vi "Update_Attribute_Tree_POLARIS.vi"(4 "Flush Tree?":bool, 5 "error in":errorcluster, 6 "Filter":string, 7 "Tree Control In":refnum<vi>, 8 "Attribute Information Array":T1[](array[typedef])) -> (0 "error out":errorcluster)   [LabVIEW 2020, in "Camera Settings Dialog UI.lvlib" / "Camera Settings Dialog.lvclass"]
doc: "The Update Attribute Tree subVI, enumerates the attributes available for the camera and populates the Attribute Tree control with the attribute list."
uses:
  Camera Settings Dialog.lvclass
  Camera Attribute Info.ctl
  Camera Settings Dialog.lvclass/Camera Settings Dialog.ctl
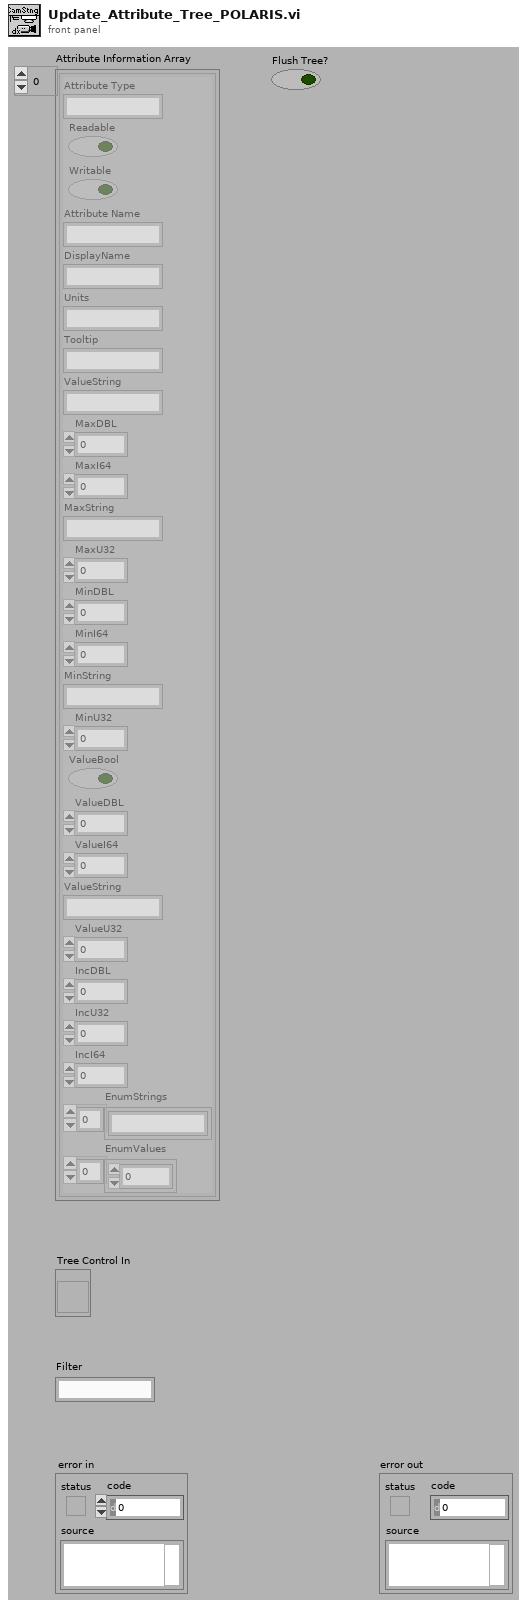
[diagram p1: front panel]
types:
  T1 = typedef "Camera Attribute Info.ctl" = cluster{"Attribute Type":string, "Readable":bool, "Writable":bool, "Attribute Name":string, "DisplayName":string, "Units":string, "Tooltip":string, "ValueString":string, "MaxDBL":dbl, "MaxI64":i64, "MaxString":string, "MaxU32":u32, "MinDBL":dbl, "MinI64":i64, "MinString":string, "MinU32":u32, "ValueBool":bool, "ValueDBL":dbl, "ValueI64 ":i64, "ValueString":string, "ValueU32":u32, "IncDBL":dbl, "IncU32":u32, "IncI64":i64, "EnumStrings":string[], "EnumValues":u32[]}
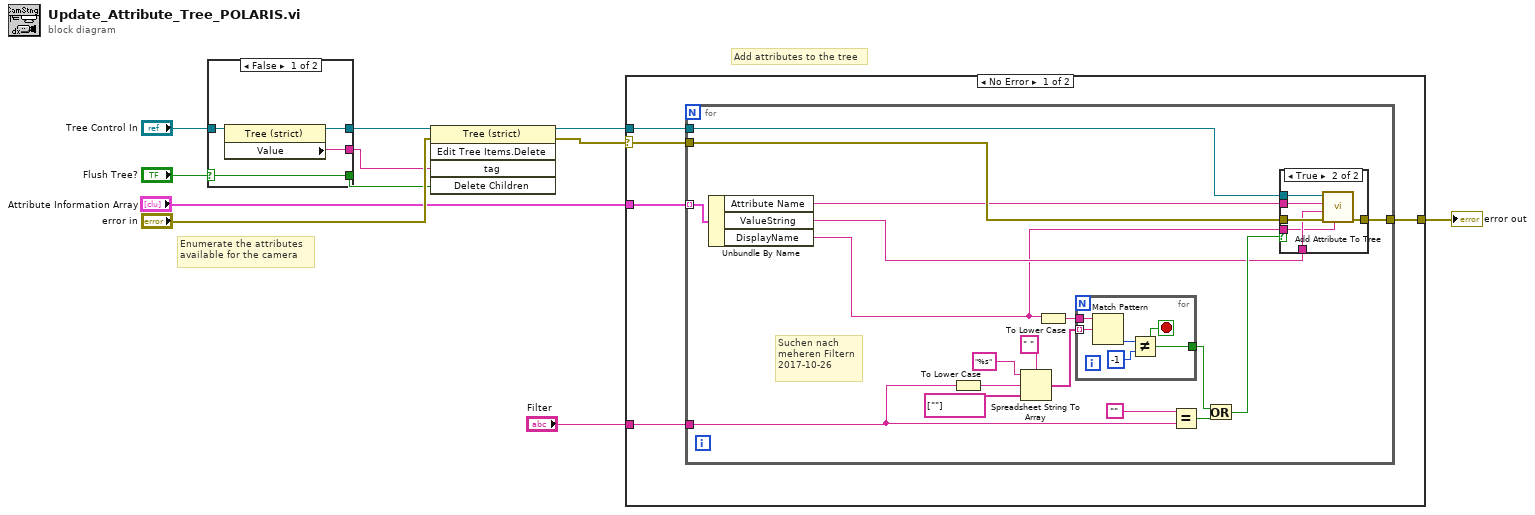
[diagram p0: block diagram]
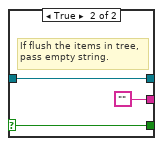
[diagram p2: hidden frame]
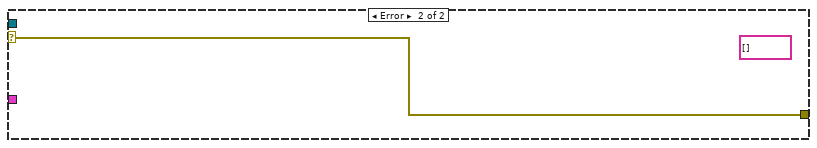
[diagram p4: hidden frame]
diagram:
  # "Add attributes to the tree"
  # "Enumerate the attributes \navailable for the camera"
  n1 = case shown="False" "Flush Tree?" {
    selector: "Flush Tree?" -> [w15 w18]
    tunnel: [w15 w18] -> w6
    tunnel: [w12 ""] -> w5
    tunnel: "Tree Control In" -> [w14 w16]
    tunnel: [w13 w16] -> w3
    frame False {
      n2 = property class="Tree (strict)"(reference=w14) -> (reference out=w13:refnum<vi>, "Value"=w12:string)  [unwired: 1 in, 1 out]
    }
    frame True {
      # "If flush the items in tree,\npass empty string."
    }
  }
  n3 = invoke class="Tree (strict)" method="Edit Tree Items.Delete"(reference=w3, error in="error in", "tag"=w5, "Delete Children"=w6) -> (reference out=w10:refnum<vi>, error out=w9:errorcluster)  [unwired: 1 in, 3 out]
  n4 = case shown="No Error" w9 {
    selector: w9 -> [w21 w54]
    tunnel: "Attribute Information Array" -> [w23 _]
    tunnel: w10 -> [w22 _]
    tunnel: [w20 w54] -> w8
    tunnel: "Filter" -> [w19 _]
    frame No Error {
      n5 = for {
        tunnel: w23 -> [w41] mode=indexing
        tunnel: w22 -> [w39]
        tunnel: w21 -> [w38]
        tunnel: [w40] -> w20
        tunnel: w19 -> [w31]
        # "Suchen nach \nmeheren Filtern\n2017-10-26"
        n6 = Unbundle By Name(w41) -> ("Attribute Name"=w36:string, "ValueString"=w25:string, "DisplayName"=w24:string)
        n7 = To Lower Case(string=w31) -> (all lower case string=w27:string)
        n8 = Spreadsheet String To Array(delimiter (Tab)=" ", format string="%s", spreadsheet string=w27, array type (2D Dbl)=string[] [""]) -> (array=w26:string[])
        n9 = To Lower Case(string=w24) -> (all lower case string=w32:string)
        n10 = for {
          tunnel: [w42] -> w34
          tunnel: w32 -> [w44]
          tunnel: w26 -> [w43] mode=indexing
          stop <- w42 stop-if-true
          n11 = Match Pattern(string=w44, regular expression=w43) -> (offset past match=w46:i32)  [unwired: 1 in, 3 out]
          n12 = Not Equal?(x=w46, y=-1) -> (x != y?=w42:bool)
        }
        n13 = Equal?(x="", y=w31) -> (x = y?=w35:bool)
        n14 = Or(x=w34, y=w35) -> (x .or. y?=w33:bool)
        n15 = case shown="True" w33 {
          tunnel: [w47 w53] -> w40
          tunnel: w39 -> [_ w52]
          tunnel: w38 -> [w47 w51]
          tunnel: w25 -> [_ w50]
          tunnel: w36 -> [_ w49]
          tunnel: w24 -> [_ w48]
          frame False {
          }
          frame True {
            n16 = call "Add Attribute To Tree.vi"("Display Name"=w48, "error in"=w51, "Value"=w50, "Attribute Name"=w49, "Attribute Table In"=w52) -> ("error out"=w53:errorcluster)  [unwired: 5 in, 1 out]
          }
        }
      }
    }
    frame Error {
      (unwired) string[] []
    }
  }
  "error out" <- w8
